vi "DELETETest Prefilters.vi"() -> ()   [LabVIEW 2019]
uses:
  Instrument.DAQ.lvclass
  Instrument.DAQ.lvclass/Instrument.DAQ.ctl
  <vilib>/measure/maspectr.llb/FFT Power Spectrum and PSD for N Chan.vi
  <vilib>/measure/NI_MAPro.lvlib
  C:/Program Files/National Instruments/LabVIEW 2019/vi.lib/JKI/JKI SMO/SMO/SMO.lvclass
  <vilib>/measure/maspectr.llb/FFT Power Spectrum and PSD for 1 Chan.vi
panel:
  out "Magnitude Response 2":cluster{"f0":dbl, "df":dbl, "magnitude":dbl[]}(graph)
  out "Magnitude Response":cluster{"f0":dbl, "df":dbl, "magnitude":dbl[]}[](graph)
  out "AI Graph 2":waveform(dbl)[](graph)
  in  "AI Graph":waveform(dbl)[](graph)
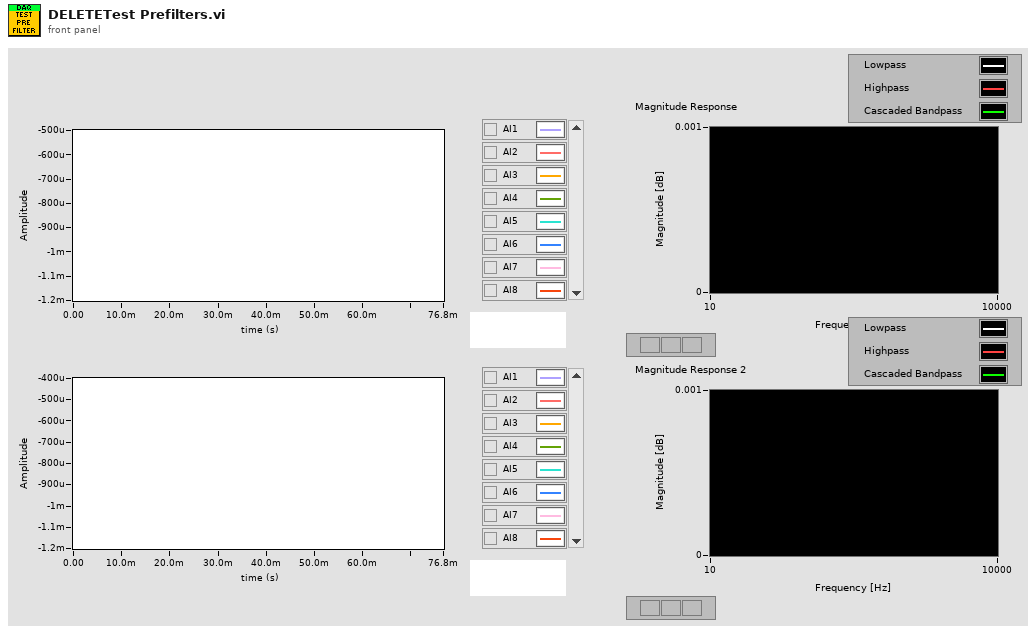
[diagram p1: front panel]
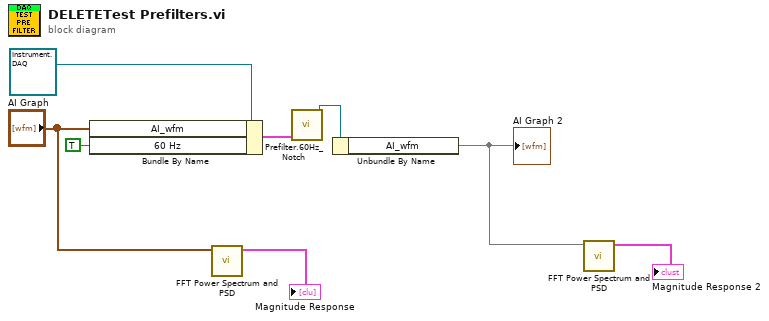
[diagram p0: block diagram]
diagram:
  n1 = Bundle By Name(cluster=refnum<class "Instrument.DAQ.lvclass"> refnum ("Instrument.DAQ"), "AI_wfm"="AI Graph", "60 Hz"=TRUE ("Configuration.Prefilter.60 Hz")) -> (w7:cluster{})
  n2 = call-poly <vilib>:"FFT Power Spectrum and PSD.vi"("time signals"="AI Graph") -> ("Power Spectrum / PSD"=→"Magnitude Response":cluster{"f0":dbl, "df":dbl, "magnitude":dbl[]}[])  [unwired: 7 in, 3 out]
  n3 = call "Prefilter.60Hz_Notch.vi"("Instrument.DAQ"=w7) -> ("Instrument.DAQ out"=w5:refnum<class "Instrument.DAQ.lvclass">)  [unwired: 9 in, 1 out]
  n4 = Unbundle By Name(w5) -> ("AI_wfm"=w3)
  "AI Graph 2" <- w3
  n5 = call-poly <vilib>:"FFT Power Spectrum and PSD.vi"("time signal"=w3) -> ("Power Spectrum / PSD"=→"Magnitude Response 2":cluster{"f0":dbl, "df":dbl, "magnitude":dbl[]})  [unwired: 7 in, 3 out]
